vi "Export Configuration RTM.vi"(8 "error in":errorcluster, 11 "Node Ptr":u64 format="%.0x") -> (0 "error out":errorcluster)   [LabVIEW 2024, in "AIM ARINC 429 System Explorer.lvlib" / "Implementation.lvlib"]
uses:
  Implementation.lvlib
  Scripting/AIM/AIM ARINC 429 Scripting.lvlib
panel:
  in  "Tag":string
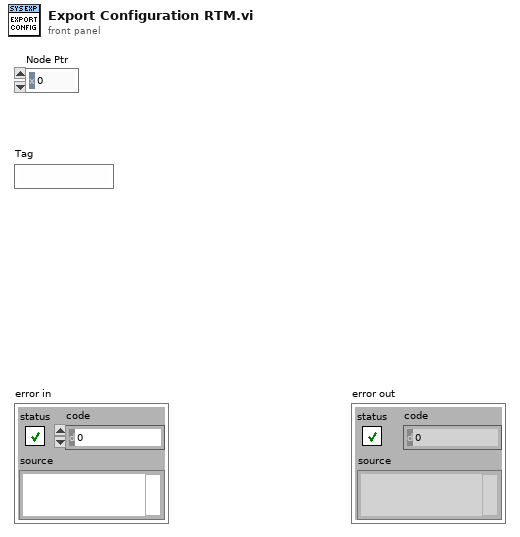
[diagram p1: front panel]
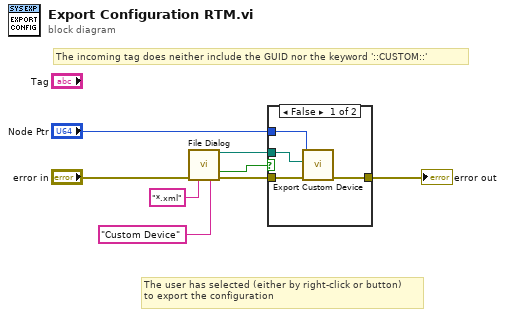
[diagram p0: block diagram]
diagram:
  # "The user has selected (either by right-click or button)\nto export the configuration"
  # "The incoming tag does neither include the GUID nor the keyword '::CUSTOM::'"
  n1 = call "File Dialog"("error in"="error in", "pattern (all files)"="*.xml" ("pattern label"), "pattern label"="Custom Device") -> ("selected path"=w3:path, "cancelled"=w5:bool, "error out"=w4:errorcluster)  [unwired: 9 in, 1 out]
  n2 = case shown="False" w5 {
    tunnel: w4 -> [w12 w13]
    tunnel: w3 -> [w11 _]
    tunnel: "Node Ptr" -> [w10 _]
    tunnel: [w9 w13] -> w1
    frame False {
      n3 = call "Export Custom Device.vi"("error in"=w12, "path"=w11, "custom device ref"=w10) -> ("error out"=w9:errorcluster)  [unwired: 7 in, 1 out]
    }
    frame True {
    }
  }
  "error out" <- w1
